vi "BRig_Host__Loop_Consumer_RunState__closedLoop_parseOutput2.vi"(5 "String":string) -> (4 "output_cmd":bool, 6 "output_cmdList":u16[][](array[numeric]), 8 "output_thres":bool, 10 "output_thres1":u16, 15 "output_thres2":u16)   [LabVIEW 2014]
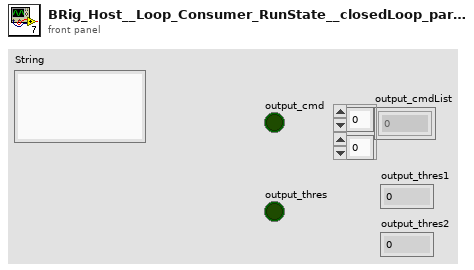
[diagram p1: front panel]
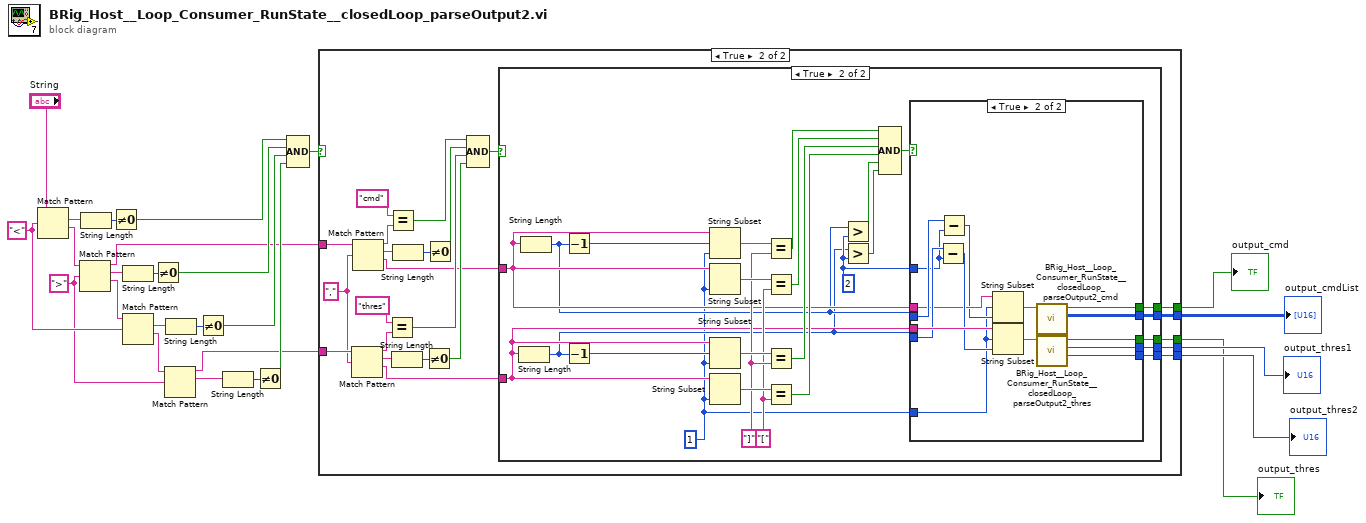
[diagram p0: block diagram]
diagram:
  w6 = ">" ("regular expression")
  w7 = "<" ("regular expression")
  n1 = Match Pattern(string="String", regular expression=w7) -> (match substring=w25:string, after substring=w21:string)  [unwired: 1 in, 2 out]
  n2 = Match Pattern(string=w21, regular expression=w6) -> (before substring=w9:string, match substring=w23:string, after substring=w18:string)  [unwired: 1 in, 1 out]
  n3 = String Length(string=w25) -> (length=w24:i32)
  n4 = Not Equal To 0?(x=w24) -> (x != 0?=w11:bool)
  n5 = String Length(string=w23) -> (length=w22:i32)
  n6 = Match Pattern(string=w18, regular expression=w7) -> (match substring=w20:string, after substring=w15:string)  [unwired: 1 in, 2 out]
  n7 = Not Equal To 0?(x=w22) -> (x != 0?=w12:bool)
  n8 = Match Pattern(string=w15, regular expression=w6) -> (before substring=w8:string, match substring=w17:string)  [unwired: 1 in, 2 out]
  n9 = String Length(string=w20) -> (length=w19:i32)
  n10 = Not Equal To 0?(x=w19) -> (x != 0?=w13:bool)
  n11 = String Length(string=w17) -> (length=w16:i32)
  n12 = Not Equal To 0?(x=w16) -> (x != 0?=w14:bool)
  n13 = Compound Arithmetic op=AND(w11, w12, w13, w14) -> (w10:bool)
  n14 = case shown="True" w10 {
    tunnel: w9 -> [_ w47]
    tunnel: w8 -> [_ w40]
    tunnel: [_ w31] -> w4
    tunnel: [_ w30] -> w3
    tunnel: [_ w29] -> w5
    tunnel: [_ w28] -> w2
    tunnel: [_ w27] -> w1
    frame False {
    }
    frame True {
      w39 = "," ("regular expression")
      n15 = Match Pattern(string=w40, regular expression=w39) -> (before substring=w42:string, match substring=w44:string, after substring=w32:string)  [unwired: 1 in, 1 out]
      n16 = Match Pattern(string=w47, regular expression=w39) -> (before substring=w46:string, match substring=w49:string, after substring=w33:string)  [unwired: 1 in, 1 out]
      n17 = Equal?(x="thres", y=w42) -> (x = y?=w37:bool)
      n18 = Equal?(x="cmd", y=w46) -> (x = y?=w35:bool)
      n19 = String Length(string=w44) -> (length=w43:i32)
      n20 = String Length(string=w49) -> (length=w48:i32)
      n21 = Not Equal To 0?(x=w43) -> (x != 0?=w38:bool)
      n22 = Not Equal To 0?(x=w48) -> (x != 0?=w36:bool)
      n23 = Compound Arithmetic op=AND(w35, w36, w37, w38) -> (w34:bool)
      n24 = case shown="True" w34 {
        tunnel: w33 -> [_ w63]
        tunnel: w32 -> [_ w64]
        tunnel: [_ w54] -> w31
        tunnel: [_ w53] -> w30
        tunnel: [_ w52] -> w29
        tunnel: [_ w51] -> w28
        tunnel: [_ w50] -> w27
        frame False {
        }
        frame True {
          w60 = 2 ("y")
          w71 = "]" ("y")
          w70 = "[" ("y")
          w55 = 1 ("length (rest)")
          n25 = String Length(string=w64) -> (length=w57:i32)
          n26 = String Length(string=w63) -> (length=w59:i32)
          n27 = Decrement(x=w59) -> (x-1=w58:i32)
          n28 = Decrement(x=w57) -> (x-1=w56:i32)
          n29 = String Subset(string=w63, offset (0)=w58, length (rest)=w55) -> (substring=w75:string)
          n30 = String Subset(string=w63, length (rest)=w55) -> (substring=w74:string)  [unwired: 1 in]
          n31 = String Subset(string=w64, offset (0)=w56, length (rest)=w55) -> (substring=w73:string)
          n32 = String Subset(string=w64, length (rest)=w55) -> (substring=w72:string)  [unwired: 1 in]
          n33 = Equal?(x=w75, y=w71) -> (x = y?=w66:bool)
          n34 = Equal?(x=w74, y=w70) -> (x = y?=w67:bool)
          n35 = Equal?(x=w73, y=w71) -> (x = y?=w68:bool)
          n36 = Equal?(x=w72, y=w70) -> (x = y?=w69:bool)
          n37 = Greater?(x=w59, y=w60) -> (0:w62:bool)
          n38 = Greater?(x=w57, y=w60) -> (0:w61:bool)
          n39 = Compound Arithmetic op=AND(w66, w67, w68, w69, w62, w61) -> (w65:bool)
          n40 = case shown="True" w65 {
            tunnel: w64 -> [_ w90]
            tunnel: w63 -> [_ w85]
            tunnel: w57 -> [_ w89]
            tunnel: w59 -> [_ w88]
            tunnel: w60 -> [_ w87]
            tunnel: w55 -> [_ w83]
            tunnel: [_ w80] -> w54
            tunnel: [_ w79] -> w53
            tunnel: [_ w78] -> w52
            tunnel: [_ w77] -> w51
            tunnel: [_ w76] -> w50
            frame False {
            }
            frame True {
              n41 = Subtract(x=w89, y=w87) -> (x-y=w86:i32)
              n42 = Subtract(x=w88, y=w87) -> (x-y=w84:i32)
              n43 = String Subset(string=w85, offset (0)=w83, length (rest)=w84) -> (substring=w81:string)
              n44 = String Subset(string=w90, offset (0)=w83, length (rest)=w86) -> (substring=w82:string)
              n45 = call "BRig_Host__Loop_Consumer_RunState__closedLoop_parseOutput2_cmd.vi"("String"=w81) -> (2:"output_cmdList"=w78:u16[][], 3:"output_cmdList"=w76:bool)  [unwired: 9 in]
              n46 = call "BRig_Host__Loop_Consumer_RunState__closedLoop_parseOutput2_thres.vi"("String"=w82) -> ("output_thres2"=w79:u16, "output_thres1"=w80:u16, "output_thres"=w77:bool)  [unwired: 8 in]
            }
          }
        }
      }
    }
  }
  "output_cmdList" <- w5
  "output_thres1" <- w4
  "output_thres2" <- w3
  "output_thres" <- w2
  "output_cmd" <- w1
